vi "Get Joystick 2013.vi"() -> (3 "Robot Controls":T1)   [LabVIEW 2014]
uses:
  SubSystems/Robot Controls.ctl
  Global Variables/Global Variables.vi
  <vilib>/Rock Robotics/WPI/Joystick/WPI_JoystickGetSetRefNum.vi
  <vilib>/Rock Robotics/Network Tables/SD Write Numeric Array.vi
  <vilib>/Rock Robotics/Network Tables/SD Write Boolean Array.vi
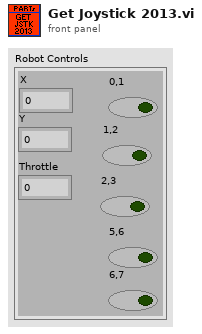
[diagram p1: front panel]
types:
  T1 = typedef "Robot Controls.ctl" = cluster{"X":dbl, "Y ":dbl, "Throttle":dbl, "0,1":bool, "1,2":bool, "2,3":bool, "5,6":bool, "6,7 ":bool}
  T2 = typedef "WPI_JoystickDevRef.ctl" = cluster{"Device":T3}
  T3 = typedef "WPI_JoystickDeviceEnum.ctl" = enum16{"USB 0", "USB 1", "USB 2", "USB 3", "USB 4", "USB 5"}
  T4 = cluster{"Axes[0]":dbl, "Axes[1]":dbl, "Axes[2]":dbl, "Axes[3]":dbl, "Axes[4]":dbl, "Axes[5]":dbl, "Axes[6]":dbl, "Axes[7]":dbl, "Axes[8]":dbl}
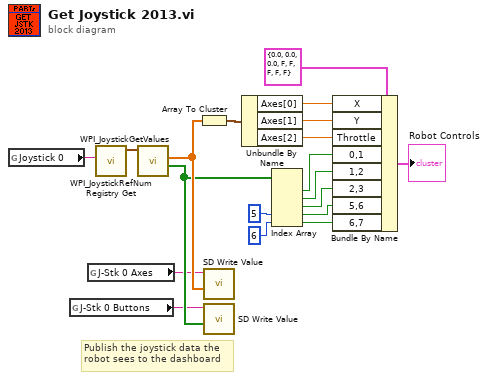
[diagram p0: block diagram]
diagram:
  # "Publish the joystick data the\nrobot sees to the dashboard"
  n1 = global read "Global Variables.vi" "Joystick 0"() -> (w19:string)
  n2 = global read "Global Variables.vi" "J-Stk 0 Buttons"() -> (w5:string)
  n3 = global read "Global Variables.vi" "J-Stk 0 Axes"() -> (w6:string)
  n4 = call <vilib>:"WPI_JoystickRefNum Registry Get.vi"("refnum name"=w19) -> ("JoystickDevRef"=w18:T2)  [unwired: 1 in, 9 out]
  n5 = call <vilib>:"WPI_JoystickGetValues.vi"("JoystickDevRef"=w18) -> ("Buttons"=w15:bool[], "Axes"=w17:dbl[])  [unwired: 6 in, 3 out]
  n6 = Array To Cluster(array=w17) -> (cluster=w16:T4)
  n7 = call-poly <vilib>:"SD Write Value.vi"("Numeric Array"=w17, "Name"=w6) -> ()  [unwired: 8 in, 2 out]
  n8 = call-poly <vilib>:"SD Write Value.vi"("Boolean Array"=w15, "Name"=w5) -> ()  [unwired: 8 in, 2 out]
  n9 = Unbundle By Name(w16) -> ("Axes[0]"=w14:dbl, "Axes[1]"=w13:dbl, "Axes[2]"=w12:dbl)
  n10 = Index Array(array=w15, index #4=5 ("index"), index #5=6 ("index")) -> (element #1=w11:bool, element #2=w10:bool, element #3=w9:bool, element #4=w2:bool, element #5=w1:bool)  [unwired: 3 in]
  n11 = Bundle By Name(cluster=T1 {"X"=0.0, "Y "=0.0, "Throttle"=0.0, "0,1"=FALSE, "1,2"=FALSE, "2,3"=FALSE, "5,6"=FALSE, "6,7 "=FALSE} ("Robot Controls"), "X"=w14, "Y"=w13, "Throttle"=w12, "0,1"=w11, "1,2"=w10, "2,3"=w9, "5,6"=w2, "6,7"=w1) -> (→"Robot Controls":T1)
